vi "Arieh Temp (Arieh Kisos's conflicted copy 2017-06-07).vi"() -> ()   [LabVIEW 2015]
uses:
  <vilib>/FPGAPlugInAG/cRIO-9030/niLvFpga_Open_cRIO-9030.vi
  <vilib>/rvi/interface/common/dynamic/niFpgaDynamicAddResources.vi
  <vilib>/FPGAPlugInAG/Dynamic/niLvFpga_Run_Dynamic.vi
  <vilib>/rvi/interface/nirviOpenFPGA/nirviOpenFPGA.xnode
  FPGA Bitfiles/BELKINEAGLEGUI_FPGATarget_EagleFPGAScanner_AddXN+PC+cM.lvbitx
  Eagle_FPGA Scanner Control.vi
  <vilib>/rvi/interface/nirviMethod/nirviMethod.xnode
panel:
  in  "Y Multi":dbl format="%#_13g"
  in  "Y Offs":dbl format="%#_13g"
  out "Y":dbl[](array[numeric])
  out "X":dbl[](array[numeric])
  in  "X Offs":dbl format="%#_13g"
  in  "X Multi":dbl format="%#_13g"
  out "PY":fxp<+,10,10>[](array[numeric])
  out "PX":fxp<+,10,10>[](array[numeric])
  in  "Radius B":fxp<+/-,10,10>=250.0
  in  "Radius A":fxp<+/-,10,10>=250.0
  in  "Center":T1={"CX"=400.0, "CY"=300.0}
types:
  T1 = cluster{"CX":fxp<+/-,10,10>, "CY":fxp<+/-,10,10>}
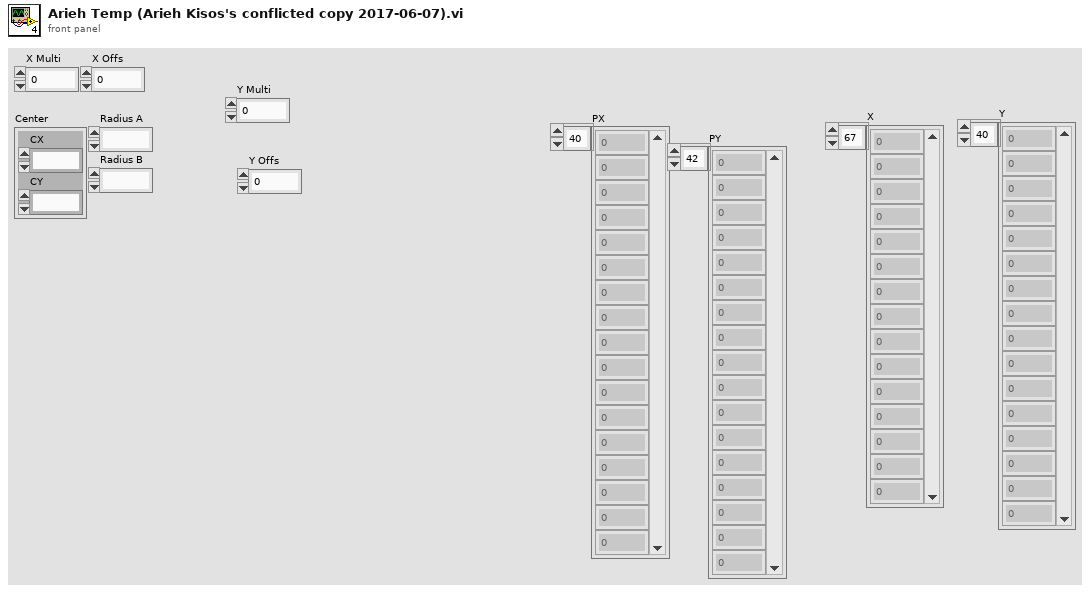
[diagram p1: front panel]
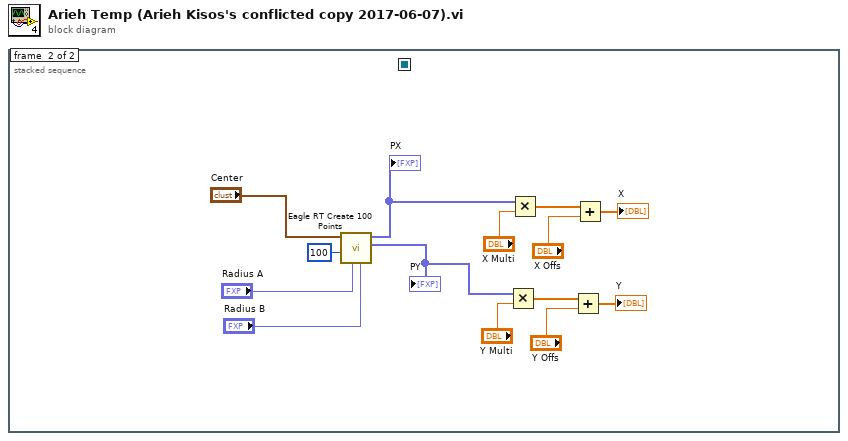
[diagram p0: block diagram]
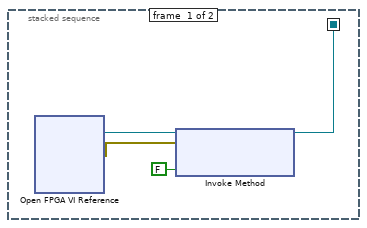
[diagram p2: hidden frame]
diagram:
  n1 = stacked-sequence {
    seq-local: [w1 _] -> [_ _]
    frame #0 {
      n2 = xnode "Open FPGA VI Reference"() -> ("FPGA VI Reference Out"=w4:refnum<k20>, "error out"=w3:errorcluster)  [unwired: 2 in]
      n3 = xnode "Invoke Method"("FPGA VI Reference In"=w4, "error in"=w3, "Wait Until Done (F)"=FALSE) -> ("FPGA VI Reference Out"=w1:refnum<k20>)  [unwired: 1 out]
    }
    frame #1 {
      n4 = call "Eagle RT Create 100 Points.vi"("Radius B"="Radius B", "Radius A"="Radius A", "NumOfPoints"=100, "Center"="Center") -> ("PY"=w5:fxp<+,10,10>[], "PX"=w14:fxp<+,10,10>[])  [unwired: 6 in]
      "PX" <- w14
      "PY" <- w5
      n5 = Multiply(x=w5, y="Y Multi") -> (x*y=w6:dbl[])
      n6 = Multiply(x=w14, y="X Multi") -> (x*y=w13:dbl[])
      n7 = Add(x=w6, y="Y Offs") -> (x+y=→"Y":dbl[])
      n8 = Add(x=w13, y="X Offs") -> (x+y=→"X":dbl[])
    }
  }
